vi "CreateMutateData.vi"(0 "LVClassLibrary Ref":refnum<vi>, 1 "New BlueSerializableVersion":u16, 5 "Application":refnum<vi>, 7 "SerializableData.ctl path":path, 9 "SerializableData_v2.ctl":path, 11 "error in (no error)":errorcluster, 12 "Mutate_Template.vi path":path, 13 "Mutate_SaveTo_Path":path) -> (4 "LVClassLibrary Ref":refnum<vi>, 6 "Application":refnum<vi>, 15 "error out":errorcluster)   [LabVIEW 2019, in "BlueSerializationScripts.lvlib"]
uses:
  BlueSerializationScripts.lvlib
  BlueSerialVirtualFolders.ctl
  BlueUtilityScripts/BlueUtilityScripts.lvlib
  <vilib>/LabVIEW Icon API/LabVIEW Icon API.lvlib
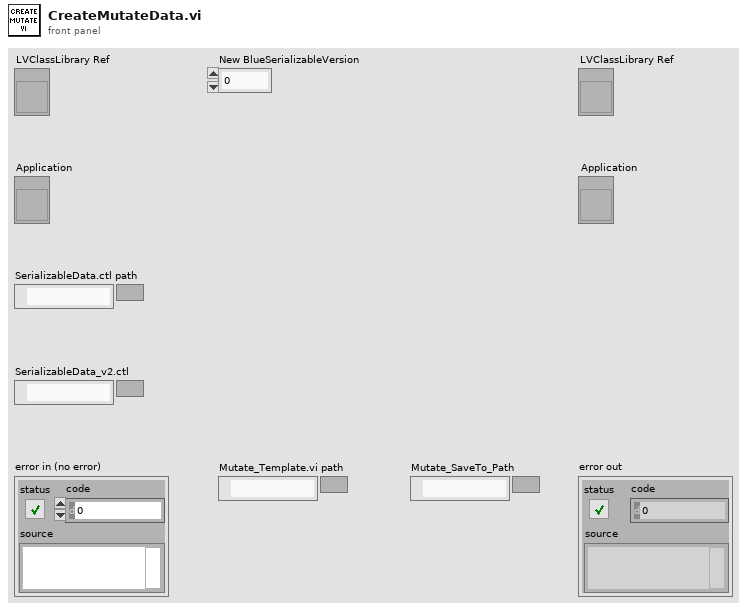
[diagram p1: front panel]
types:
  T1 = typedef "BlueSerializationScripts.lvlib/BlueSerialVirtualFolders.ctl" = enum16{"BlueSerialization", "Mutations"}
  T2 = enum32{"invalid VI type", "Standard VI", "Control VI", "Global VI", "Polymorphic VI", "Configuration VI", "SubSystem", "Facade VI", "Method VI"}
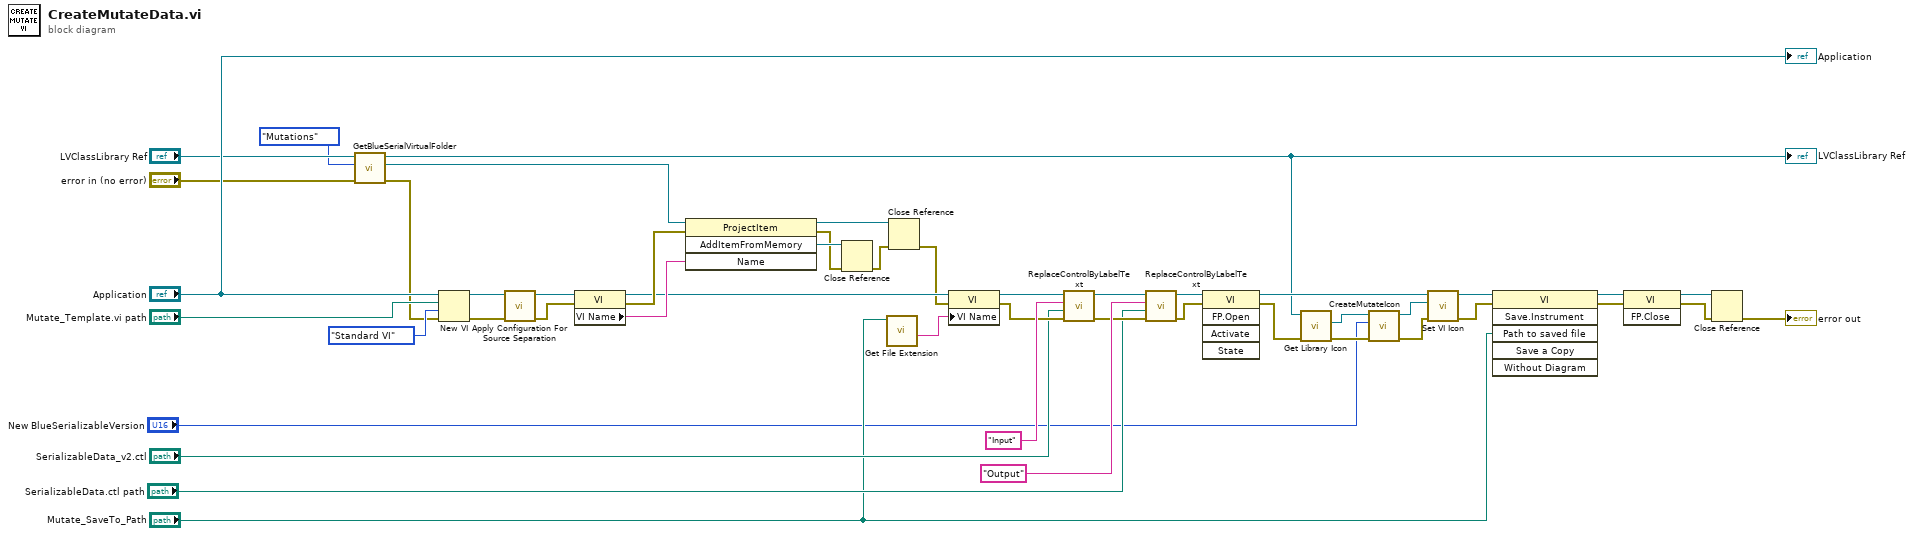
[diagram p0: block diagram]
diagram:
  n1 = call "GetBlueSerialVirtualFolder.vi"("error in (no error)"="error in (no error)", "Virtual Folder"=BlueSerialVirtualFolders."Mutations", "LVClassLibrary Ref"="LVClassLibrary Ref") -> ("error out"=w23:errorcluster, "Folder Refnum out"=w22:refnum<vi>, "LVClassLibrary Ref"=w3:refnum<vi>)  [unwired: 6 in]
  "LVClassLibrary Ref" <- w3
  n2 = New VI(8:w23, 9:T2."Standard VI" ("vi type (standard vi)"), 10:"Mutate_Template.vi path", 11:"Application") -> (0:w29:errorcluster, 3:w30:refnum<vi>)  [unwired: 3 out]
  n3 = call <vilib>:"Apply Configuration For Source Separation.vi"("error in (no error)"=w29, "VI in"=w30) -> ("error out"=w33:errorcluster, "VI out"=w35:refnum<vi>)  [unwired: 8 in]
  n4 = property class="VI"(reference=w35, error in=w33) -> (reference out=w36:refnum<vi>, error out=w38:errorcluster, "VI Name"=w37:string)
  n5 = invoke class="ProjectItem" method="AddItemFromMemory"(reference=w22, error in=w38, "Name"=w37) -> (reference out=w31:refnum<vi>, error out=w26:errorcluster, "AddItemFromMemory"=w27:refnum<vi>)  [unwired: 1 in, 1 out]
  n6 = Close Reference(reference=w27, error in (no error)=w26) -> (error out=w25:errorcluster)
  n7 = call <vilib>:"Get File Extension.vi"("file"="Mutate_SaveTo_Path") -> ("filename without extension"=w34:string)  [unwired: 6 in, 4 out]
  n8 = Close Reference(reference=w31, error in (no error)=w25) -> (error out=w32:errorcluster)
  n9 = property class="VI"(reference=w36, error in=w32, "VI Name"=w34) -> (reference out=w21:refnum<vi>, error out=w19:errorcluster)
  n10 = call "ReplaceControlByLabelText.vi"("error in (no error)"=w19, "Replacement Path"="SerializableData_v2.ctl", "Control Label.text"="Input", "VI ref"=w21) -> ("error out"=w16:errorcluster, "VI ref"=w18:refnum<vi>)  [unwired: 5 in, 1 out]
  n11 = call "ReplaceControlByLabelText.vi"("error in (no error)"=w16, "Replacement Path"="SerializableData.ctl path", "Control Label.text"="Output", "VI ref"=w18) -> ("error out"=w11:errorcluster, "VI ref"=w12:refnum<vi>)  [unwired: 5 in, 1 out]
  n12 = invoke class="VI" method="FP.Open"(reference=w12, error in=w11) -> (reference out=w8:refnum<vi>, error out=w5:errorcluster)  [unwired: 3 in, 3 out]
  n13 = call <vilib>:"Get Library Icon.vi"("error in (no error)"=w5, "Library Refnum in"=w3) -> ("error out"=w4:errorcluster, "Icon"=w1:refnum<class "Icon.lvclass">)  [unwired: 7 in, 1 out]
  n14 = call "CreateMutateIcon.vi"("error in (no error)"=w4, "New BlueSerializableVersion"="New BlueSerializableVersion", "Icon.lvclass in"=w1) -> ("error out"=w10:errorcluster, "Icon.lvlclass out"=w9:refnum<class "Icon.lvclass">)  [unwired: 6 in, 1 out]
  n15 = call <vilib>:"Set VI Icon.vi"("error in (no error)"=w10, "Icon"=w9, "VI Refnum in"=w8) -> ("error out"=w6:errorcluster, "VI Refnum out"=w7:refnum<vi>)  [unwired: 7 in]
  n16 = invoke class="VI" method="Save.Instrument"(reference=w7, error in=w6, "Path to saved file"="Mutate_SaveTo_Path") -> (reference out=w42:refnum<vi>, error out=w41:errorcluster)  [unwired: 3 in, 4 out]
  n17 = invoke class="VI" method="FP.Close"(reference=w42, error in=w41) -> (reference out=w40:refnum<vi>, error out=w39:errorcluster)  [unwired: 1 in, 1 out]
  n18 = Close Reference(reference=w40, error in (no error)=w39) -> (error out=→"error out":errorcluster)
  "Application" <- "Application"
